vi "proba_z_subvi.vi"() -> ()   [LabVIEW 2020]
panel:
  in  "stop":bool
  out "password 2":string
  out "login 2":string
  out "Time":string
  out "Date":string
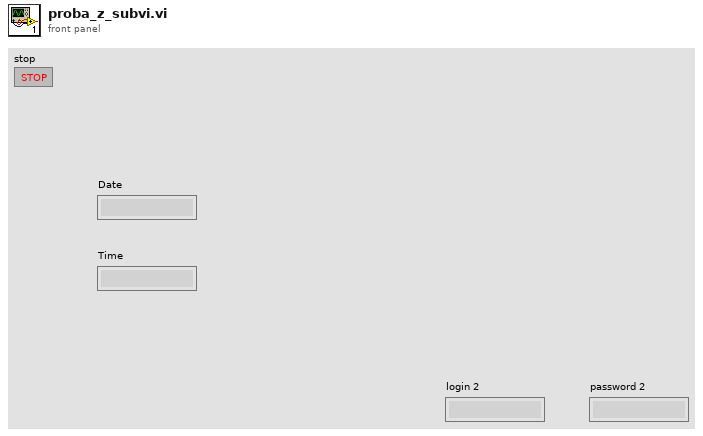
[diagram p1: front panel]
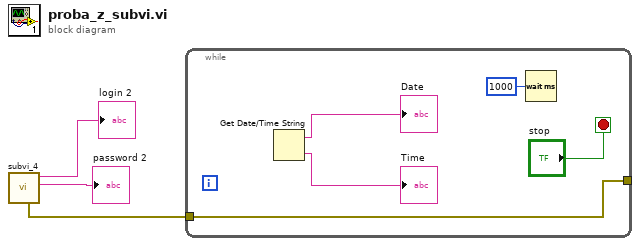
[diagram p0: block diagram]
diagram:
  n1 = call "subvi_4.vi"() -> ("password out"=→"password 2":string, "login out"=→"login 2":string, "error out"=w1:errorcluster)  [unwired: 9 in]
  n2 = while {
    tunnel: w1 -> [w5]
    tunnel: [w5] -> _
    stop <- "stop" stop-if-true
    n3 = Get Date/Time String() -> (date string=→"Date":string, time string=→"Time":string)  [unwired: 3 in]
    n4 = Wait (ms)(milliseconds to wait=u32 1000) -> ()  [unwired: 1 out]
  }
